vi "Icon Edit Test.vi"() -> ()   [LabVIEW 2014]
uses:
  Initialization Scripting/Icon Editor/Icon Editor.llb/Icon Colors.ctl
  Initialization Scripting/Initialization and IO Node Scripting.lvlib
panel:
  out "Error Out":errorcluster
  in  "Icon Text":string="AI 0"
  in  "Icon Colors":T1={"Text Color"=0, "Background Color"=16448250, "Border Color"=16746744}
  in  "Error In":errorcluster
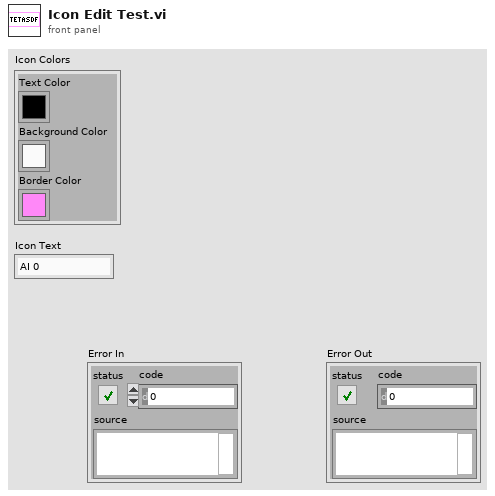
[diagram p1: front panel]
types:
  T1 = typedef "Initialization and IO Node Scripting.lvlib/Icon Colors.ctl" = cluster{"Text Color":u32, "Background Color":u32, "Border Color":u32}
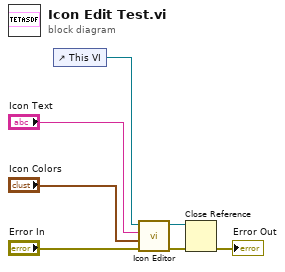
[diagram p0: block diagram]
diagram:
  n1 = control-ref of="This VI"() -> (w1:refnum<vi>)
  n2 = call "Icon Editor.vi"("Error In"="Error In", "Icon Colors"="Icon Colors", "Icon Text"="Icon Text", "Reference to VI"=w1) -> ("Error Out"=w4:errorcluster, "Reference to VI"=w3:refnum<vi>)  [unwired: 6 in]
  n3 = Close Reference(reference=w3, error in (no error)=w4) -> (error out=→"Error Out":errorcluster)
